vi "Create Reference.vi"(10 "uid":string, 11 "class":string) -> (3 "Reference":refnum<class "Reference.lvclass">)   [LabVIEW 2020, in "VILab.lvlib" / "Reference.lvclass"]
uses:
  Reference.lvclass
  C:/Users/User/Documents/LabVIEW Data/Projects/VILab/source/SubVIs/Classes/Element/Element.lvclass
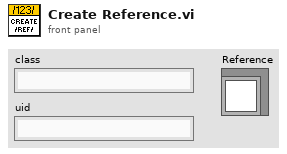
[diagram p1: front panel]
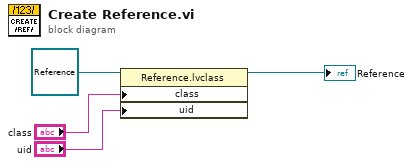
[diagram p0: block diagram]
diagram:
  n1 = property class="Reference.lvclass"(reference=refnum<class "Reference.lvclass"> refnum ("VILab.lvlib:Reference.lvclass"), "class"="class", "uid"="uid") -> (reference out=→"Reference":refnum<class "Reference.lvclass">)  [unwired: 1 in, 1 out]
